vi "startEnobio.vi"(8 "error in (no error)":errorcluster, 11 "address":string="127.0.0.1") -> (0 "error out":errorcluster, 3 "connection ID":refnum<k5>)   [LabVIEW 2013]
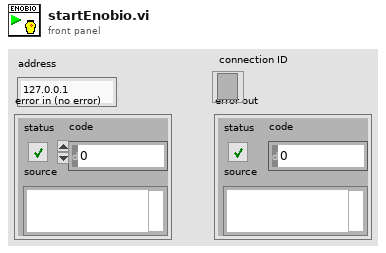
[diagram p1: front panel]
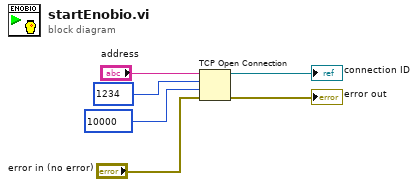
[diagram p0: block diagram]
diagram:
  n1 = TCP Open Connection(address="address", remote port or service name=u16 1234, timeout ms (60000)=10000, error in (no error)="error in (no error)") -> (connection ID=→"connection ID":refnum<k5>, error out=→"error out":errorcluster)  [unwired: 1 in]
